vi "Save_Ensight_Case.vi"() -> (5 "Plug in titles":string[](array[string]), 7 "Plug in values":string[](array[string]))   [LabVIEW 2020]
uses:
  Globals/Meas_global.vi
  <vilib>/Analysis/NI_AALBase.lvlib
  <vilib>/Analysis/baseanly.llb/Mean (DBL).vi
panel:
  out "Z":dbl
  out "Y":dbl
  out "X":dbl
  out "Channel Varaibles":string[](array[string])
  out "Variable Names":string[](array[string])
  out "File Paths":path[](array[path])
  out "Results Folder Exists?":bool
  # "You must have just these two indicators on the connector pane of the vi"
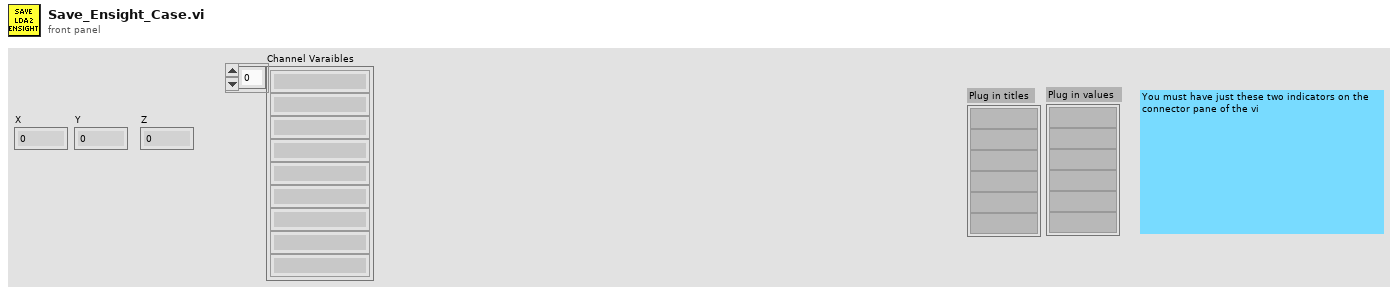
[diagram p1: front panel]
types:
  T1 = typedef "Analysis_info_cluster.ctl" = cluster{"Colour":u32, "Inst type":T2, "Inst name":string, "Symbol":string, "Code name":string, "Extra Info":string, "Inst Array":T3, "Extra Titles":string[], "Extra Values":string[], "U":dbl, "u^2":dbl, "u^3":dbl, "u^4":dbl, "Skew_u":dbl, "Kurt_u":dbl, "Sd Error in Mean":dbl, "% u'/U":dbl, "X":dbl, "Y":dbl, "Z":dbl, "Timescale integral Estimate":dbl, "Sd Error in Variance":dbl, "Calib File":path, "Calib Constants":dbl[], "Output Position":bool, "Stats":enum16{"None", "Basic", "Full"}, "Av Sampling Rate":dbl, "Av No of Samples":dbl, "Total Meas Time (s)":dbl, "ADAM Ch Name":string, "Max value":dbl, "Min value":dbl, "Req Sample Rate Hz":dbl, "Sync Delay Time (s)":dbl, "Ch No":i16, "Device":string, "Use Latest Calib":bool, "Port":string, "Metadata Ch Names":string[], "Metadata Ch Values":string[], "Label":string}
  T2 = typedef "Inst_type.ctl" = enum16{"Propeller anemometer", "Raw voltage", "Pressure Transducer", "Pitot-static tube", "Hot wire", "Cross wire 1", "Cross wire 2", "Generic Linear", "Generic Polynomial", "Generic BackPoly", "Fast FID", "Thermocouple", "Cold wire", "Pulsed Wire", "LDA Vel", "LDA Tran time", "LDA Arr time", "Microphone"}
  T3 = typedef "Instrument_Array.ctl" = enum16{"PWA", "LDA", "Analogue"}
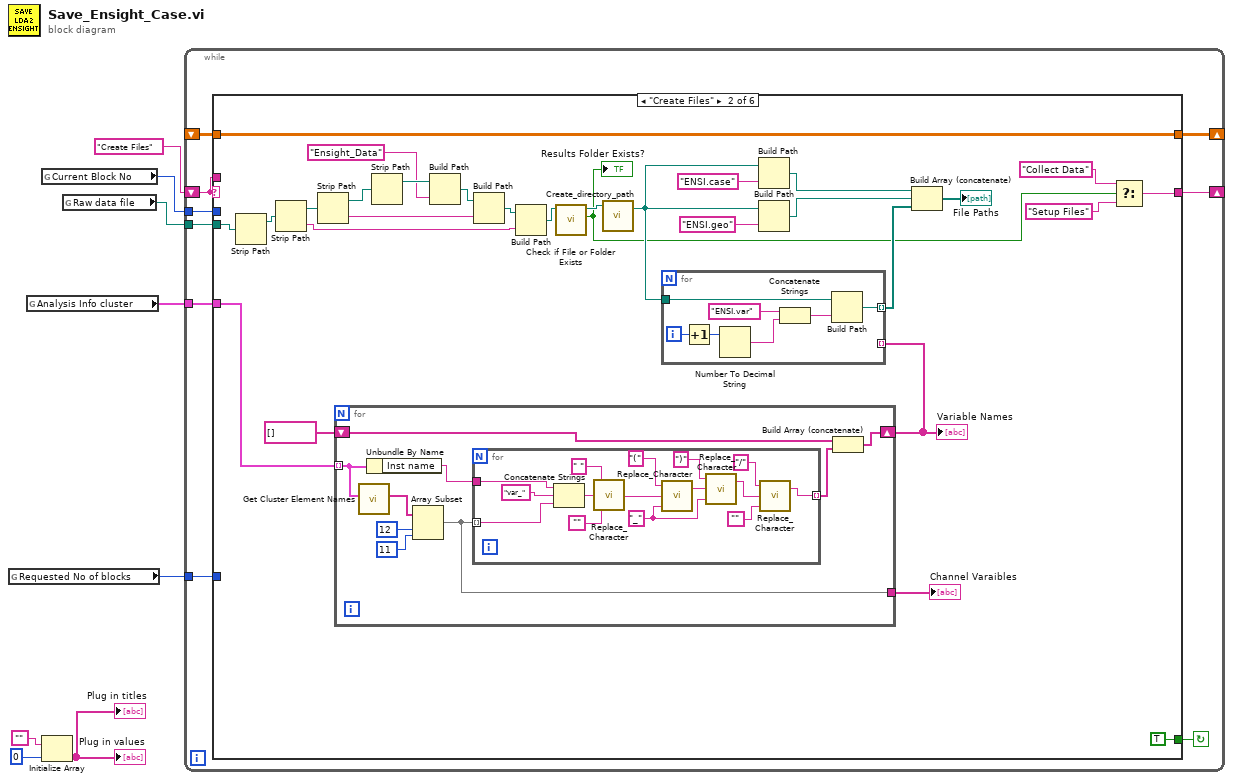
[diagram p0: block diagram]
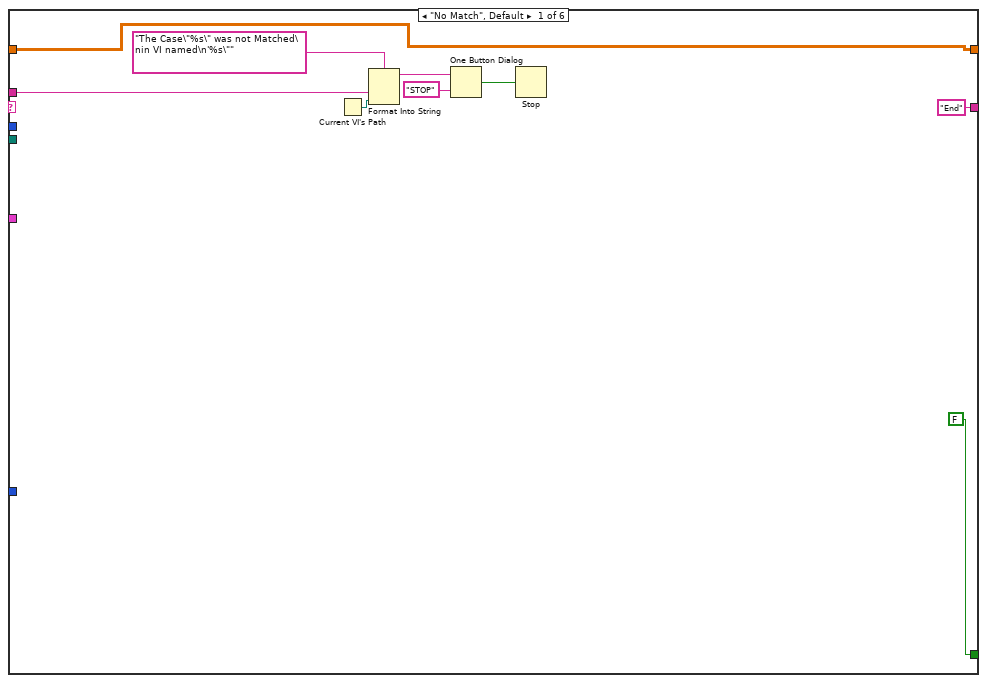
[diagram p2: hidden frame]
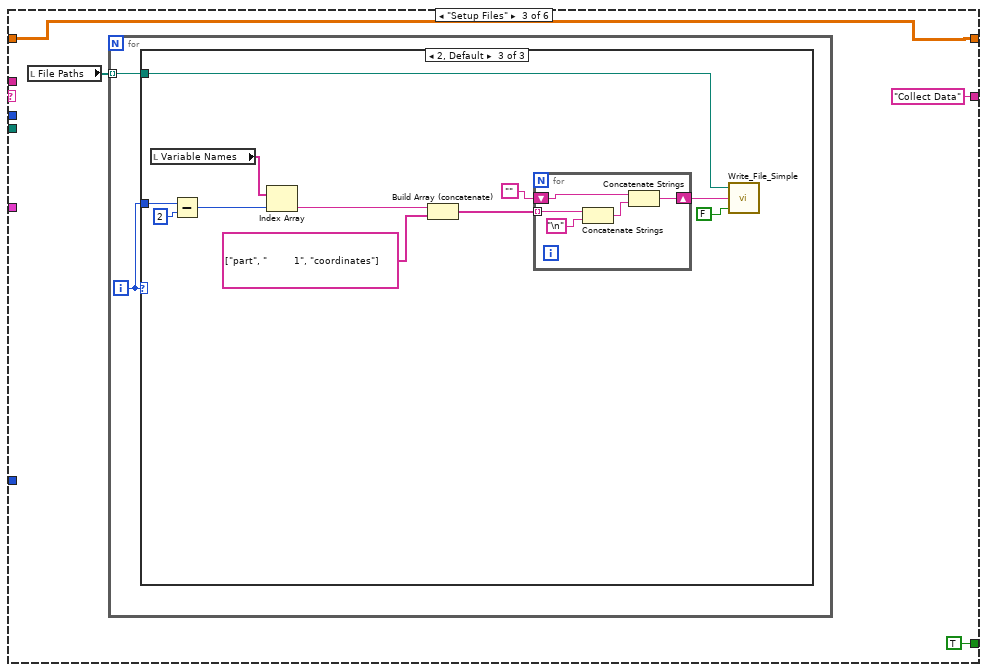
[diagram p3: hidden frame]
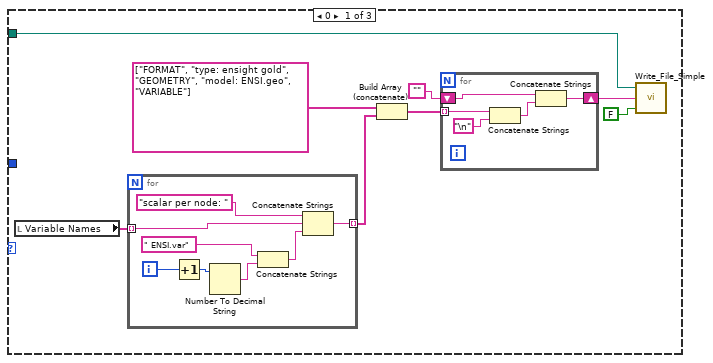
[diagram p4: hidden frame]
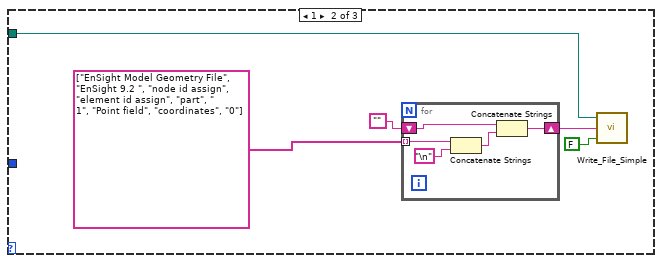
[diagram p5: hidden frame]
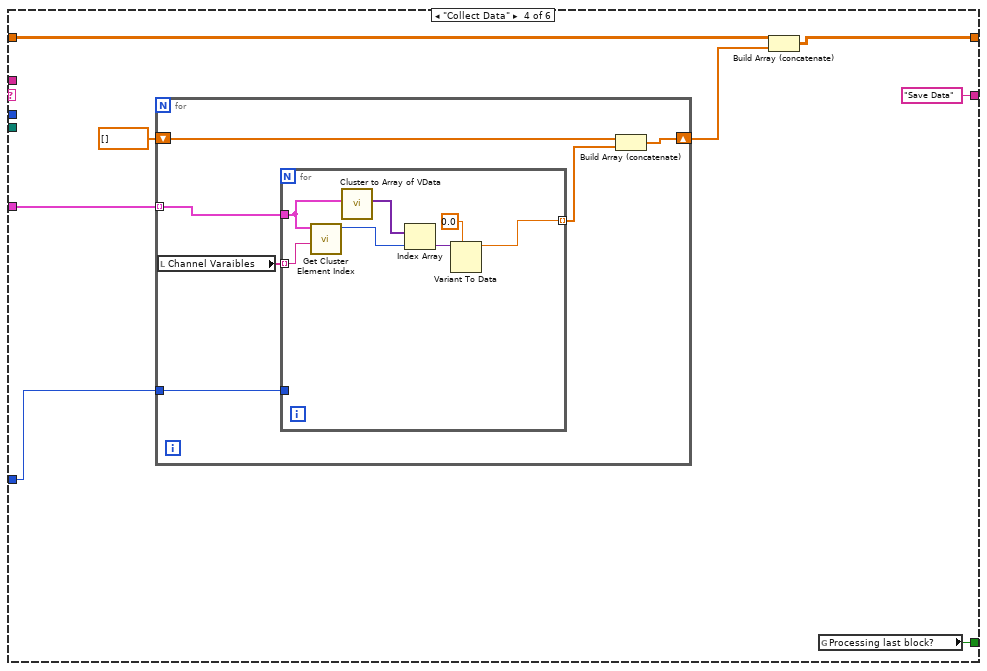
[diagram p6: hidden frame]
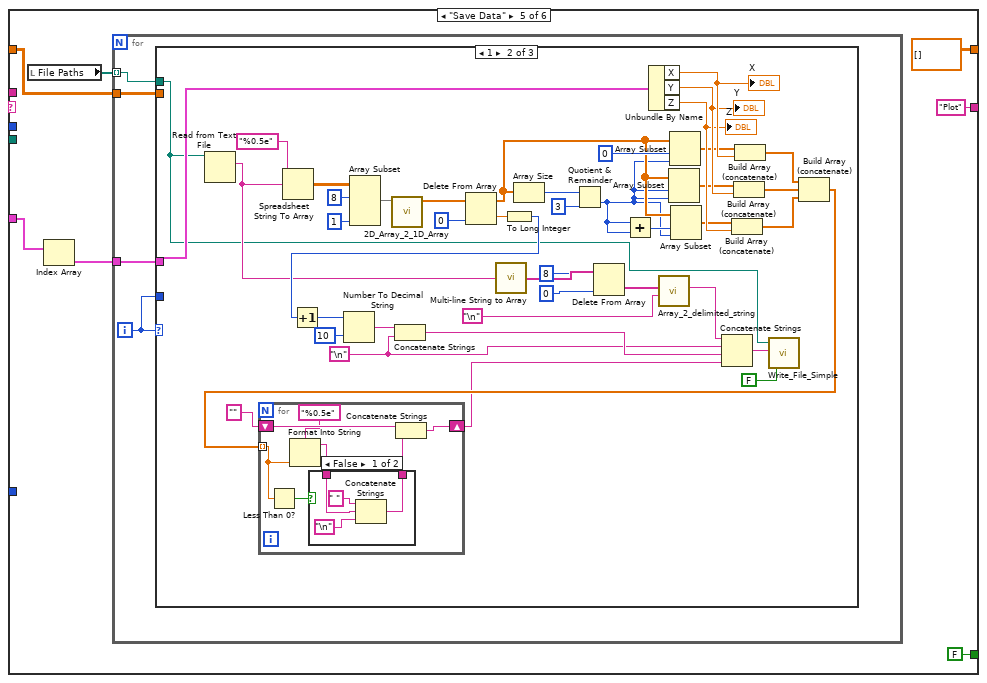
[diagram p7: hidden frame]
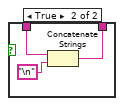
[diagram p9: hidden frame]
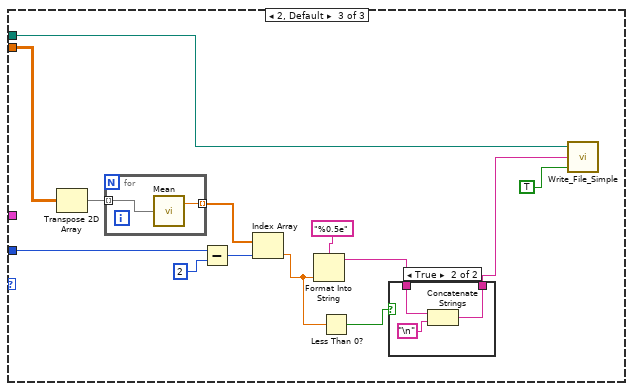
[diagram p10: hidden frame]
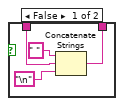
[diagram p11: hidden frame]
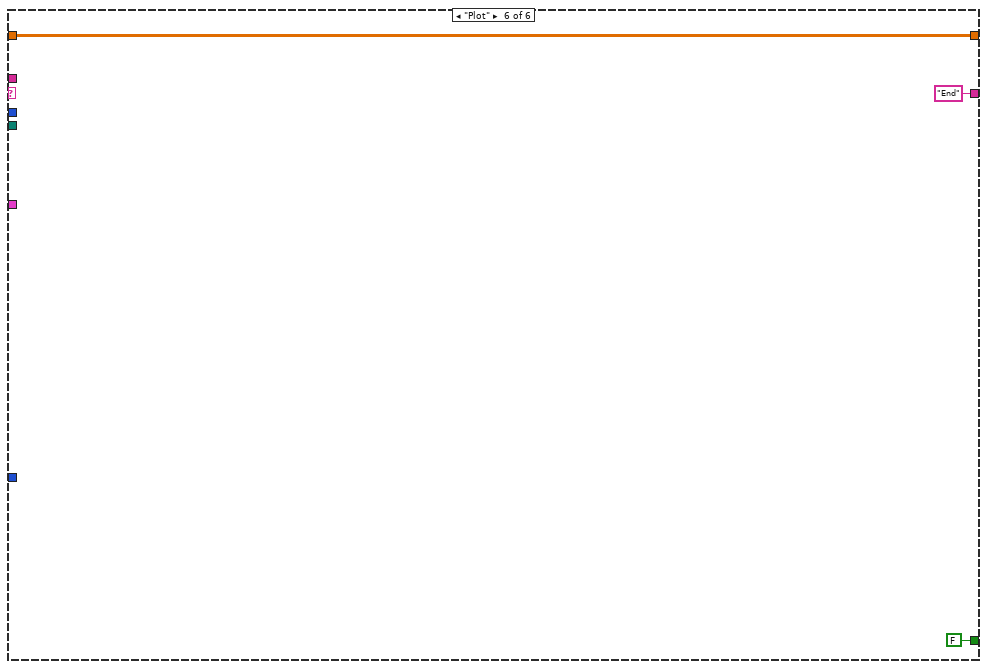
[diagram p12: hidden frame]
diagram:
  n1 = global read "Meas_global.vi" "Requested No of blocks"() -> (w1:i32)
  n2 = global read "Meas_global.vi" "Analysis Info cluster"() -> (w2:T1[])
  n3 = global read "Meas_global.vi" "Current Block No"() -> (w4:i32)
  n4 = Initialize Array("", 0) -> (→"Plug in values" →"Plug in titles":string[])
  n5 = global read "Meas_global.vi" "Raw data file"() -> (w3:path)
  n6 = while {
    shift-left: "Create Files" -> [w17]
    shift-right: [w16] -> _
    tunnel: w4 -> [w14]
    tunnel: w3 -> [w13]
    tunnel: w2 -> [w12]
    tunnel: w1 -> [w11]
    shift-right: [w10] -> _
    shift-left: _ -> [w9]
    stop <- w15 continue-if-true
    n7 = case shown="\"Create Files\"" w17 {
      tunnel: ["End" ("t") w38 "Collect Data" ("t") "Save Data" ("t") "Plot" ("t") "End" ("t")] -> w16
      tunnel: w17 -> [w22 _ _ _ _ _]
      tunnel: [FALSE TRUE ("Processing last block?") TRUE ("Processing last block?") w147 FALSE ("Processing last block?") FALSE ("Processing last block?")] -> w15
      tunnel: w14 -> [_ _ _ _ _ _]
      tunnel: w13 -> [_ w55 _ _ _ _]
      tunnel: w12 -> [_ w34 _ w146 w161 _]
      tunnel: w11 -> [_ _ _ w145 _ _]
      tunnel: [w18 w27 w87 w141 dbl[][] [] w251] -> w10
      tunnel: w9 -> [w18 w27 w87 w140 w162 w251]
      frame "No Match", Default {
        n8 = Current VI's Path() -> (path=w21:path)
        n9 = Format Into String(format string="The Case\"%s\" was not Matched\nin VI named\n'%s\"" ("Format String"), w22, w21) -> (resulting string=w25:string)  [unwired: 2 in, 1 out]
        n10 = One Button Dialog(message=w25, button name ("OK")="STOP") -> (true=w23:bool)
        n11 = Stop(stop? (T)=w23) -> ()
      }
      frame "Create Files" {
        n12 = Strip Path(path=w55) -> (stripped path=w54:path)  [unwired: 1 out]
        n13 = Strip Path(path=w54) -> (stripped path=w53:path, name=w28:string)
        n14 = Strip Path(path=w53) -> (stripped path=w52:path, name=w48:string)
        n15 = for {
          tunnel: w34 -> [w56] mode=indexing
          shift-right: [w60] -> w31
          shift-left: string[] [] -> [w58]
          tunnel: [w57] -> w32
          n16 = call "Get Cluster Element Names.vi"("Cluster"=w56) -> ("Element Names"=w64:string[])  [unwired: 9 in, 1 out]
          n17 = Unbundle By Name(w56) -> ("Inst name"=w61:string)
          n18 = Array Subset(array=w64, index=12, length=11) -> (w57:string[])
          n19 = for {
            tunnel: w57 -> [w79] mode=indexing
            tunnel: w61 -> [w78]
            tunnel: [w66] -> w59 mode=indexing
            w70 = "_" ("Replace with")
            n20 = Concatenate Strings(w78, "var_" ("string"), w79) -> (w76:string)
            n21 = call "Replace_Character.vi"("Replace with"="", "Input String"=w76, "Search For"=" ") -> ("Output string"=w65:string)  [unwired: 1 out]
            n22 = call "Replace_Character.vi"("Replace with"=w70, "Input String"=w65, "Search For"="(") -> ("Output string"=w72:string)  [unwired: 1 out]
            n23 = call "Replace_Character.vi"("Replace with"=w70, "Input String"=w72, "Search For"=")") -> ("Output string"=w69:string)  [unwired: 1 out]
            n24 = call "Replace_Character.vi"("Replace with"="", "Input String"=w69, "Search For"="/") -> ("Output string"=w66:string)  [unwired: 1 out]
          }
          n25 = Build Array (concatenate)(w58, w59) -> (w60:string[])
        }
        "Variable Names" <- w31
        "Channel Varaibles" <- w32
        n26 = Strip Path(path=w52) -> (stripped path=w51:path)  [unwired: 1 out]
        n27 = Build Path(base path=w51, name or relative path="Ensight_Data") -> (appended path=w49:path)
        n28 = Build Path(base path=w49, name or relative path=w48) -> (appended path=w29:path)
        n29 = Build Path(base path=w29, name or relative path=w28) -> (appended path=w30:path)
        n30 = call <vilib>:"Check if File or Folder Exists.vi"("path"=w30) -> ("file or folder exists?"=w37:bool, "dup path"=w47:path)  [unwired: 8 in, 1 out]
        "Results Folder Exists?" <- w37
        n31 = call "Create_directory_path.vi"("Path name"=w47) -> ("Path name Out"=w43:path)  [unwired: 2 in, 1 out]
        n32 = for {
          tunnel: w43 -> [w86]
          tunnel: [w80] -> w40 mode=indexing
          tunnel: w31 -> [_] mode=indexing
          i -> [w85]
          n33 = Increment(x=w85) -> (x+1=w84:i32)
          n34 = Number To Decimal String(number=w84) -> (decimal integer string=w82:string)  [unwired: 1 in]
          n35 = Concatenate Strings("ENSI.var" ("name or relative path"), w82) -> (w81:string)
          n36 = Build Path(base path=w86, name or relative path=w81) -> (appended path=w80:path)
        }
        n37 = Build Path(base path=w43, name or relative path="ENSI.case") -> (appended path=w42:path)
        n38 = Build Path(base path=w43, name or relative path="ENSI.geo") -> (appended path=w41:path)
        n39 = Build Array (concatenate)(w42, w41, w40) -> (→"File Paths":path[])
        n40 = Select(t="Collect Data", s=w37, f="Setup Files" ("t")) -> (s? t:f=w38:string)
      }
      frame "Setup Files" {
        n41 = local read "File Paths"() -> (w89:path[])
        n42 = for {
          tunnel: w89 -> [w92] mode=indexing
          i -> [w91]
          n43 = case shown="2, Default" w91 {
            tunnel: w92 -> [w96 w115 w134]
            tunnel: w91 -> [_ _ w129]
            frame 0 {
              n44 = local read "Variable Names"() -> (w100:string[])
              n45 = for {
                tunnel: w100 -> [w108] mode=indexing
                tunnel: [w106] -> w94 mode=indexing
                i -> [w111]
                n46 = Increment(x=w111) -> (x+1=w112:i32)
                n47 = Number To Decimal String(number=w112) -> (decimal integer string=w109:string)  [unwired: 1 in]
                n48 = Concatenate Strings(" ENSI.var", w109) -> (w107:string)
                n49 = Concatenate Strings("scalar per node: ", w108, w107) -> (w106:string)
              }
              n50 = Build Array (concatenate)(string[] ["FORMAT", "type: ensight gold", "GEOMETRY", "model: ENSI.geo", "VARIABLE"], w94) -> (w93:string[])
              n51 = for {
                tunnel: w93 -> [w105] mode=indexing
                shift-right: [w103] -> w98
                shift-left: "" -> [w101]
                n52 = Concatenate Strings(w105, "\n") -> (w102:string)
                n53 = Concatenate Strings(w101, w102) -> (w103:string)
              }
              n54 = call "Write_File_Simple.vi"("append to file? (new file:F)"=FALSE, "character string"=w98, "file path"=w96) -> ()  [unwired: 2 out]
            }
            frame 1 {
              n55 = for {
                tunnel: string[] ["EnSight Model Geometry File", "EnSight 9.2 ", "node id assign", "element id assign", "part", "         1", "Point field", "coordinates", "0"] -> [w123] mode=indexing
                shift-right: [w121] -> w117
                shift-left: "" -> [w119]
                n56 = Concatenate Strings(w123, "\n") -> (w120:string)
                n57 = Concatenate Strings(w119, w120) -> (w121:string)
              }
              n58 = call "Write_File_Simple.vi"("append to file? (new file:F)"=FALSE, "character string"=w117, "file path"=w115) -> ()  [unwired: 2 out]
            }
            frame 2, Default {
              n59 = local read "Variable Names"() -> (w130:string[])
              n60 = Subtract(x=w129, y=2) -> (x-y=w127:i32)
              n61 = Index Array(array=w130, index=w127) -> (element=w126:string)
              n62 = Build Array (concatenate)(w126, string[] ["part", "         1", "coordinates"]) -> (w124:string[])
              n63 = for {
                tunnel: w124 -> [w139] mode=indexing
                shift-right: [w137] -> w132
                shift-left: "" -> [w135]
                n64 = Concatenate Strings(w139, "\n") -> (w136:string)
                n65 = Concatenate Strings(w135, w136) -> (w137:string)
              }
              n66 = call "Write_File_Simple.vi"("append to file? (new file:F)"=FALSE, "character string"=w132, "file path"=w134) -> ()  [unwired: 2 out]
            }
          }
        }
      }
      frame "Collect Data" {
        n67 = for {
          tunnel: w146 -> [w152] mode=indexing
          tunnel: w145 -> [w153]
          shift-right: [w149] -> w142
          shift-left: dbl[] [] -> [w150]
          n68 = local read "Channel Varaibles"() -> (w151:string[])
          n69 = for {
            tunnel: w153 -> [_]
            tunnel: w152 -> [w158]
            tunnel: w151 -> [w160] mode=indexing
            tunnel: [w154] -> w148 mode=indexing
            n70 = call "Get Cluster Element Index.vi"("Element Name"=w160, "Cluster"=w158) -> ("Element Index"=w159:i32)  [unwired: 9 in]
            n71 = call "Cluster to Array of VData.vi"("Cluster"=w158) -> ("Array of VData"=w157:variant[])  [unwired: 9 in, 1 out]
            n72 = Index Array(array=w157, index=w159) -> (element=w156:variant)
            n73 = Variant To Data(type=0.0, Variant=w156) -> (data=w154:dbl)  [unwired: 1 in, 1 out]
          }
          n74 = Build Array (concatenate)(w150, w148) -> (w149:dbl[])
        }
        n75 = Build Array (concatenate)(w140, w142) -> (w141:dbl[][])
        n76 = global read "Meas_global.vi" "Processing last block?"() -> (w147:bool)
      }
      frame "Save Data" {
        n77 = local read "File Paths"() -> (w165:path[])
        n78 = Index Array(array=w161) -> (element=w164:T1)  [unwired: 1 in]
        n79 = for {
          tunnel: w165 -> [w171] mode=indexing
          tunnel: w164 -> [w170]
          tunnel: w162 -> [w168]
          i -> [w169]
          n80 = case shown="1" w169 {
            tunnel: w171 -> [_ w172 w241]
            tunnel: w170 -> [_ w208 _]
            tunnel: w169 -> [_ _ w240]
            tunnel: w168 -> [_ _ w236]
            frame 0 {
            }
            frame 1 {
              w190 = "\n"
              n81 = Read from Text File(file (use dialog)=w172) -> (text=w205:string)  [unwired: 3 in, 3 out]
              n82 = Spreadsheet String To Array(format string="%0.5e", spreadsheet string=w205) -> (array=w209:dbl[][])  [unwired: 2 in]
              n83 = Array Subset(array=w209, index (row)=8 ("index"), length (col)=1 ("length")) -> (w212:dbl[][])  [unwired: 2 in]
              n84 = call "2D_Array_2_1D_Array.vi"("Array in"=w212) -> ("Array out"=w213:dbl[])  [unwired: 10 in]
              n85 = Delete From Array(array=w213, index=0) -> (deleted portion=w186:dbl, array with subset deleted=w178:dbl[])  [unwired: 1 in]
              n86 = call "Multi-line String to Array.vi"("Multi lined string"=w205) -> ("Array of string lines"=w204:string[])
              n87 = To Long Integer(number=w186) -> (32bit integer=w207:i32)
              n88 = Increment(x=w207) -> (x+1=w201:i32)
              n89 = Number To Decimal String(number=w201, width (-)=i16 10) -> (decimal integer string=w200:string)
              n90 = Concatenate Strings(w200, w190) -> (w191:string)
              n91 = Array Size(array=w178) -> (size(s)=w181:i32)
              n92 = Quotient & Remainder(x=w181, y=3) -> (floor(x/y)=w176:i32)  [unwired: 1 out]
              n93 = Delete From Array(array=w204, length=8 ("index"), index=0) -> (deleted portion=w188:string[])  [unwired: 1 out]
              n94 = Add(x=w176, y=w176) -> (x+y=w177:i32)
              n95 = Unbundle By Name(w208) -> ("X"=w197:dbl, "Y"=w196:dbl, "Z"=w195:dbl)
              "X" <- w197
              "Y" <- w196
              "Z" <- w195
              n96 = call "Array_2_delimited_string.vi"("delimiter (Tab)"="\n", "Array of Strings"=w188) -> ("delimited string"=w187:string)  [unwired: 9 in]
              n97 = Array Subset(array=w178, index=w176, length=w176) -> (w174:dbl[])
              n98 = Array Subset(array=w178, index=0, length=w176) -> (w175:dbl[])
              n99 = Array Subset(array=w178, index=w177, length=w176) -> (w173:dbl[])
              n100 = Build Array (concatenate)(w173, w195) -> (w192:dbl[])
              n101 = Build Array (concatenate)(w174, w196) -> (w193:dbl[])
              n102 = Build Array (concatenate)(w175, w197) -> (w194:dbl[])
              n103 = Build Array (concatenate)(w194, w193, w192) -> (w185:dbl[])
              n104 = for {
                tunnel: w185 -> [w216] mode=indexing
                shift-right: [w221] -> w183
                shift-left: "" -> [w220]
                n105 = Less Than 0?(x=w216) -> (x < 0?=w215:bool)
                n106 = Format Into String(format string="%0.5e", w216) -> (resulting string=w217:string)  [unwired: 2 in, 1 out]
                n107 = case shown="False" w215 {
                  tunnel: [w223 w227] -> w219
                  tunnel: w217 -> [w224 w226]
                  frame False {
                    n108 = Concatenate Strings(" " ("string"), w224, "\n") -> (w223:string)
                  }
                  frame True {
                    n109 = Concatenate Strings(w226, "\n") -> (w227:string)
                  }
                }
                n110 = Concatenate Strings(w220, w219) -> (w221:string)
              }
              n111 = Concatenate Strings(w187, w190, w191, w183) -> (w199:string)
              n112 = call "Write_File_Simple.vi"("append to file? (new file:F)"=FALSE, "character string"=w199, "file path"=w172) -> ()  [unwired: 2 out]
            }
            frame 2, Default {
              n113 = Transpose 2D Array(2D array=w236) -> (transposed array=w234:dbl[][])
              n114 = for {
                tunnel: w234 -> [w250] mode=indexing
                tunnel: [w249] -> w235 mode=indexing
                n115 = call-poly <vilib>:"Mean.vi"("X"=w250) -> ("mean"=w249:dbl)  [unwired: 1 out]
              }
              n116 = Subtract(x=w240, y=2) -> (x-y=w238:i32)
              n117 = Index Array(array=w235, index=w238) -> (element=w230:dbl)
              n118 = Format Into String(format string="%0.5e", w230) -> (resulting string=w232:string)  [unwired: 2 in, 1 out]
              n119 = Less Than 0?(x=w230) -> (x < 0?=w229:bool)
              n120 = case shown="True" w229 {
                tunnel: [w243 w247] -> w231
                tunnel: w232 -> [w244 w246]
                frame False {
                  n121 = Concatenate Strings(" " ("string"), w244, "\n") -> (w243:string)
                }
                frame True {
                  n122 = Concatenate Strings(w246, "\n") -> (w247:string)
                }
              }
              n123 = call "Write_File_Simple.vi"("append to file? (new file:F)"=TRUE, "character string"=w231, "file path"=w241) -> ()  [unwired: 2 out]
            }
          }
        }
      }
      frame "Plot" {
      }
    }
  }
